vi "App - analyze RUS V6.vi"() -> ()   [LabVIEW 2021] (continued)
"lorentzian"={"A (VHz)"=0.0, "ω (Hz)"=0.0, "Γ (Hz)"=0.0, "φ (rad)"=0.0, "Q"=0.0, "Norm  Ampl"=0.0, "z∞ (V)"=0.0+0.0i, "4corners"={"z (-pi/2)"=0.0+0.0i, "z(inf)"=0.0+0.0i, "z (pi/2)"=0.0+0.0i, "z center"=0.0+0.0i, "z(0)"=0.0+0.0i, "radius"=0.0}}, "timestamp(min)"=1735.7333333343267, "timestamp"=timestamp(3493831965 s since 1904-01-01), "Magn Field(T)"=0.0}, {"temperature"=32.55, "lorentzian"={"A (VHz)"=0.0, "ω (Hz)"=0.0, "Γ (Hz)"=0.0, "φ (rad)"=0.0, "Q"=0.0, "Norm  Ampl"=0.0, "z∞ (V)"=0.0+0.0i, "4corners"={"z (-pi/2)"=0.0+0.0i, "z(inf)"=0.0+0.0i, "z (pi/2)"=0.0+0.0i, "z center"=0.0+0.0i, "z(0)"=0.0+0.0i, "radius"=0.0}}, "timestamp(min)"=1737.0500000044703, "timestamp"=timestamp(3493832044 s since 1904-01-01), "Magn Field(T)"=0.0}, {"temperature"=32.462, "lorentzian"={"A (VHz)"=0.0, "ω (Hz)"=0.0, "Γ (Hz)"=0.0, "φ (rad)"=0.0, "Q"=0.0, "Norm  Ampl"=0.0, "z∞ (V)"=0.0+0.0i, "4corners"={"z (-pi/2)"=0.0+0.0i, "z(inf)"=0.0+0.0i, "z (pi/2)"=0.0+0.0i, "z center"=0.0+0.0i, "z(0)"=0.0+0.0i, "radius"=0.0}}, "timestamp(min)"=1738.3666666671634, "timestamp"=timestamp(3493832123 s since 1904-01-01), "Magn Field(T)"=0.0}, {"temperature"=32.371, "lorentzian"={"A (VHz)"=0.0, "ω (Hz)"=0.0, "Γ (Hz)"=0.0, "φ (rad)"=0.0, "Q"=0.0, "Norm  Ampl"=0.0, "z∞ (V)"=0.0+0.0i, "4corners"={"z (-pi/2)"=0.0+0.0i, "z(inf)"=0.0+0.0i, "z (pi/2)"=0.0+0.0i, "z center"=0.0+0.0i, "z(0)"=0.0+0.0i, "radius"=0.0}}, "timestamp(min)"=1739.7000000029802, "timestamp"=timestamp(3493832203 s since 1904-01-01), "Magn Field(T)"=0.0}, {"temperature"=32.282, "lorentzian"={"A (VHz)"=0.0, "ω (Hz)"=0.0, "Γ (Hz)"=0.0, "φ (rad)"=0.0, "Q"=0.0, "Norm  Ampl"=0.0, "z∞ (V)"=0.0+0.0i, "4corners"={"z (-pi/2)"=0.0+0.0i, "z(inf)"=0.0+0.0i, "z (pi/2)"=0.0+0.0i, "z center"=0.0+0.0i, "z(0)"=0.0+0.0i, "radius"=0.0}}, "timestamp(min)"=1741.0166666656733, "timestamp"=timestamp(3493832282 s since 1904-01-01), "Magn Field(T)"=0.0}, {"temperature"=32.189, "lorentzian"={"A (VHz)"=0.0, "ω (Hz)"=0.0, "Γ (Hz)"=0.0, "φ (rad)"=0.0, "Q"=0.0, "Norm  Ampl"=0.0, "z∞ (V)"=0.0+0.0i, "4corners"={"z (-pi/2)"=0.0+0.0i, "z(inf)"=0.0+0.0i, "z (pi/2)"=0.0+0.0i, "z center"=0.0+0.0i, "z(0)"=0.0+0.0i, "radius"=0.0}}, "timestamp(min)"=1742.3500000014901, "timestamp"=timestamp(3493832362 s since 1904-01-01), "Magn Field(T)"=0.0}, {"temperature"=32.102, "lorentzian"={"A (VHz)"=0.0, "ω (Hz)"=0.0, "Γ (Hz)"=0.0, "φ (rad)"=0.0, "Q"=0.0, "Norm  Ampl"=0.0, "z∞ (V)"=0.0+0.0i, "4corners"={"z (-pi/2)"=0.0+0.0i, "z(inf)"=0.0+0.0i, "z (pi/2)"=0.0+0.0i, "z center"=0.0+0.0i, "z(0)"=0.0+0.0i, "radius"=0.0}}, "timestamp(min)"=1743.6666666641831, "timestamp"=timestamp(3493832441 s since 1904-01-01), "Magn Field(T)"=0.0}, {"temperature"=32.008, "lorentzian"={"A (VHz)"=0.0, "ω (Hz)"=0.0, "Γ (Hz)"=0.0, "φ (rad)"=0.0, "Q"=0.0, "Norm  Ampl"=0.0, "z∞ (V)"=0.0+0.0i, "4corners"={"z (-pi/2)"=0.0+0.0i, "z(inf)"=0.0+0.0i, "z (pi/2)"=0.0+0.0i, "z center"=0.0+0.0i, "z(0)"=0.0+0.0i, "radius"=0.0}}, "timestamp(min)"=1744.9833333343267, "timestamp"=timestamp(3493832520 s since 1904-01-01), "Magn Field(T)"=0.0}, {"temperature"=31.925, "lorentzian"={"A (VHz)"=0.0, "ω (Hz)"=0.0, "Γ (Hz)"=0.0, "φ (rad)"=0.0, "Q"=0.0, "Norm  Ampl"=0.0, "z∞ (V)"=0.0+0.0i, "4corners"={"z (-pi/2)"=0.0+0.0i, "z(inf)"=0.0+0.0i, "z (pi/2)"=0.0+0.0i, "z center"=0.0+0.0i, "z(0)"=0.0+0.0i, "radius"=0.0}}, "timestamp(min)"=1746.3166666701436, "timestamp"=timestamp(3493832600 s since 1904-01-01), "Magn Field(T)"=0.0}, {"temperature"=31.83, "lorentzian"={"A (VHz)"=0.0, "ω (Hz)"=0.0, "Γ (Hz)"=0.0, "φ (rad)"=0.0, "Q"=0.0, "Norm  Ampl"=0.0, "z∞ (V)"=0.0+0.0i, "4corners"={"z (-pi/2)"=0.0+0.0i, "z(inf)"=0.0+0.0i, "z (pi/2)"=0.0+0.0i, "z center"=0.0+0.0i, "z(0)"=0.0+0.0i, "radius"=0.0}}, "timestamp(min)"=1747.6333333328366, "timestamp"=timestamp(3493832679 s since 1904-01-01), "Magn Field(T)"=0.0}, {"temperature"=31.738, "lorentzian"={"A (VHz)"=0.0, "ω (Hz)"=0.0, "Γ (Hz)"=0.0, "φ (rad)"=0.0, "Q"=0.0, "Norm  Ampl"=0.0, "z∞ (V)"=0.0+0.0i, "4corners"={"z (-pi/2)"=0.0+0.0i, "z(inf)"=0.0+0.0i, "z (pi/2)"=0.0+0.0i, "z center"=0.0+0.0i, "z(0)"=0.0+0.0i, "radius"=0.0}}, "timestamp(min)"=1748.9500000029802, "timestamp"=timestamp(3493832758 s since 1904-01-01), "Magn Field(T)"=0.0}, {"temperature"=31.653, "lorentzian"={"A (VHz)"=0.0, "ω (Hz)"=0.0, "Γ (Hz)"=0.0, "φ (rad)"=0.0, "Q"=0.0, "Norm  Ampl"=0.0, "z∞ (V)"=0.0+0.0i, "4corners"={"z (-pi/2)"=0.0+0.0i, "z(inf)"=0.0+0.0i, "z (pi/2)"=0.0+0.0i, "z center"=0.0+0.0i, "z(0)"=0.0+0.0i, "radius"=0.0}}, "timestamp(min)"=1750.2833333313465, "timestamp"=timestamp(3493832838 s since 1904-01-01), "Magn Field(T)"=0.0}, {"temperature"=31.556, "lorentzian"={"A (VHz)"=0.0, "ω (Hz)"=0.0, "Γ (Hz)"=0.0, "φ (rad)"=0.0, "Q"=0.0, "Norm  Ampl"=0.0, "z∞ (V)"=0.0+0.0i, "4corners"={"z (-pi/2)"=0.0+0.0i, "z(inf)"=0.0+0.0i, "z (pi/2)"=0.0+0.0i, "z center"=0.0+0.0i, "z(0)"=0.0+0.0i, "radius"=0.0}}, "timestamp(min)"=1751.6000000014901, "timestamp"=timestamp(3493832917 s since 1904-01-01), "Magn Field(T)"=0.0}, {"temperature"=31.463, "lorentzian"={"A (VHz)"=0.0, "ω (Hz)"=0.0, "Γ (Hz)"=0.0, "φ (rad)"=0.0, "Q"=0.0, "Norm  Ampl"=0.0, "z∞ (V)"=0.0+0.0i, "4corners"={"z (-pi/2)"=0.0+0.0i, "z(inf)"=0.0+0.0i, "z (pi/2)"=0.0+0.0i, "z center"=0.0+0.0i, "z(0)"=0.0+0.0i, "radius"=0.0}}, "timestamp(min)"=1752.933333337307, "timestamp"=timestamp(3493832997 s since 1904-01-01), "Magn Field(T)"=0.0}, {"temperature"=31.383, "lorentzian"={"A (VHz)"=0.0, "ω (Hz)"=0.0, "Γ (Hz)"=0.0, "φ (rad)"=0.0, "Q"=0.0, "Norm  Ampl"=0.0, "z∞ (V)"=0.0+0.0i, "4corners"={"z (-pi/2)"=0.0+0.0i, "z(inf)"=0.0+0.0i, "z (pi/2)"=0.0+0.0i, "z center"=0.0+0.0i, "z(0)"=0.0+0.0i, "radius"=0.0}}, "timestamp(min)"=1754.25, "timestamp"=timestamp(3493833076 s since 1904-01-01), "Magn Field(T)"=0.0}, {"temperature"=31.282, "lorentzian"={"A (VHz)"=0.0, "ω (Hz)"=0.0, "Γ (Hz)"=0.0, "φ (rad)"=0.0, "Q"=0.0, "Norm  Ampl"=0.0, "z∞ (V)"=0.0+0.0i, "4corners"={"z (-pi/2)"=0.0+0.0i, "z(inf)"=0.0+0.0i, "z (pi/2)"=0.0+0.0i, "z center"=0.0+0.0i, "z(0)"=0.0+0.0i, "radius"=0.0}}, "timestamp(min)"=1755.5666666701436, "timestamp"=timestamp(3493833155 s since 1904-01-01), "Magn Field(T)"=0.0}, {"temperature"=31.196, "lorentzian"={"A (VHz)"=0.0, "ω (Hz)"=0.0, "Γ (Hz)"=0.0, "φ (rad)"=0.0, "Q"=0.0, "Norm  Ampl"=0.0, "z∞ (V)"=0.0+0.0i, "4corners"={"z (-pi/2)"=0.0+0.0i, "z(inf)"=0.0+0.0i, "z (pi/2)"=0.0+0.0i, "z center"=0.0+0.0i, "z(0)"=0.0+0.0i, "radius"=0.0}}, "timestamp(min)"=1756.8999999985099, "timestamp"=timestamp(3493833235 s since 1904-01-01), "Magn Field(T)"=0.0}, {"temperature"=31.111, "lorentzian"={"A (VHz)"=0.0, "ω (Hz)"=0.0, "Γ (Hz)"=0.0, "φ (rad)"=0.0, "Q"=0.0, "Norm  Ampl"=0.0, "z∞ (V)"=0.0+0.0i, "4corners"={"z (-pi/2)"=0.0+0.0i, "z(inf)"=0.0+0.0i, "z (pi/2)"=0.0+0.0i, "z center"=0.0+0.0i, "z(0)"=0.0+0.0i, "radius"=0.0}}, "timestamp(min)"=1758.2166666686535, "timestamp"=timestamp(3493833314 s since 1904-01-01), "Magn Field(T)"=0.0}, {"temperature"=31.006, "lorentzian"={"A (VHz)"=0.0, "ω (Hz)"=0.0, "Γ (Hz)"=0.0, "φ (rad)"=0.0, "Q"=0.0, "Norm  Ampl"=0.0, "z∞ (V)"=0.0+0.0i, "4corners"={"z (-pi/2)"=0.0+0.0i, "z(inf)"=0.0+0.0i, "z (pi/2)"=0.0+0.0i, "z center"=0.0+0.0i, "z(0)"=0.0+0.0i, "radius"=0.0}}, "timestamp(min)"=1759.5333333313465, "timestamp"=timestamp(3493833393 s since 1904-01-01), "Magn Field(T)"=0.0}, {"temperature"=30.926, "lorentzian"={"A (VHz)"=0.0, "ω (Hz)"=0.0, "Γ (Hz)"=0.0, "φ (rad)"=0.0, "Q"=0.0, "Norm  Ampl"=0.0, "z∞ (V)"=0.0+0.0i, "4corners"={"z (-pi/2)"=0.0+0.0i, "z(inf)"=0.0+0.0i, "z (pi/2)"=0.0+0.0i, "z center"=0.0+0.0i, "z(0)"=0.0+0.0i, "radius"=0.0}}, "timestamp(min)"=1760.8666666671634, "timestamp"=timestamp(3493833473 s since 1904-01-01), "Magn Field(T)"=0.0}, {"temperature"=30.834, "lorentzian"={"A (VHz)"=0.0, "ω (Hz)"=0.0, "Γ (Hz)"=0.0, "φ (rad)"=0.0, "Q"=0.0, "Norm  Ampl"=0.0, "z∞ (V)"=0.0+0.0i, "4corners"={"z (-pi/2)"=0.0+0.0i, "z(inf)"=0.0+0.0i, "z (pi/2)"=0.0+0.0i, "z center"=0.0+0.0i, "z(0)"=0.0+0.0i, "radius"=0.0}}, "timestamp(min)"=1762.183333337307, "timestamp"=timestamp(3493833552 s since 1904-01-01), "Magn Field(T)"=0.0}, {"temperature"=30.738, "lorentzian"={"A (VHz)"=0.0, "ω (Hz)"=0.0, "Γ (Hz)"=0.0, "φ (rad)"=0.0, "Q"=0.0, "Norm  Ampl"=0.0, "z∞ (V)"=0.0+0.0i, "4corners"={"z (-pi/2)"=0.0+0.0i, "z(inf)"=0.0+0.0i, "z (pi/2)"=0.0+0.0i, "z center"=0.0+0.0i, "z(0)"=0.0+0.0i, "radius"=0.0}}, "timestamp(min)"=1763.5166666656733, "timestamp"=timestamp(3493833632 s since 1904-01-01), "Magn Field(T)"=0.0}, {"temperature"=30.648, "lorentzian"={"A (VHz)"=0.0, "ω (Hz)"=0.0, "Γ (Hz)"=0.0, "φ (rad)"=0.0, "Q"=0.0, "Norm  Ampl"=0.0, "z∞ (V)"=0.0+0.0i, "4corners"={"z (-pi/2)"=0.0+0.0i, "z(inf)"=0.0+0.0i, "z (pi/2)"=0.0+0.0i, "z center"=0.0+0.0i, "z(0)"=0.0+0.0i, "radius"=0.0}}, "timestamp(min)"=1764.8333333358169, "timestamp"=timestamp(3493833711 s since 1904-01-01), "Magn Field(T)"=0.0}, {"temperature"=30.563, "lorentzian"={"A (VHz)"=0.0, "ω (Hz)"=0.0, "Γ (Hz)"=0.0, "φ (rad)"=0.0, "Q"=0.0, "Norm  Ampl"=0.0, "z∞ (V)"=0.0+0.0i, "4corners"={"z (-pi/2)"=0.0+0.0i, "z(inf)"=0.0+0.0i, "z (pi/2)"=0.0+0.0i, "z center"=0.0+0.0i, "z(0)"=0.0+0.0i, "radius"=0.0}}, "timestamp(min)"=1766.1499999985099, "timestamp"=timestamp(3493833790 s since 1904-01-01), "Magn Field(T)"=0.0}, {"temperature"=30.467, "lorentzian"={"A (VHz)"=0.0, "ω (Hz)"=0.0, "Γ (Hz)"=0.0, "φ (rad)"=0.0, "Q"=0.0, "Norm  Ampl"=0.0, "z∞ (V)"=0.0+0.0i, "4corners"={"z (-pi/2)"=0.0+0.0i, "z(inf)"=0.0+0.0i, "z (pi/2)"=0.0+0.0i, "z center"=0.0+0.0i, "z(0)"=0.0+0.0i, "radius"=0.0}}, "timestamp(min)"=1767.4833333343267, "timestamp"=timestamp(3493833870 s since 1904-01-01), "Magn Field(T)"=0.0}, {"temperature"=30.376, "lorentzian"={"A (VHz)"=0.0, "ω (Hz)"=0.0, "Γ (Hz)"=0.0, "φ (rad)"=0.0, "Q"=0.0, "Norm  Ampl"=0.0, "z∞ (V)"=0.0+0.0i, "4corners"={"z (-pi/2)"=0.0+0.0i, "z(inf)"=0.0+0.0i, "z (pi/2)"=0.0+0.0i, "z center"=0.0+0.0i, "z(0)"=0.0+0.0i, "radius"=0.0}}, "timestamp(min)"=1768.8000000044703, "timestamp"=timestamp(3493833949 s since 1904-01-01), "Magn Field(T)"=0.0}, {"temperature"=30.285, "lorentzian"={"A (VHz)"=0.0, "ω (Hz)"=0.0, "Γ (Hz)"=0.0, "φ (rad)"=0.0, "Q"=0.0, "Norm  Ampl"=0.0, "z∞ (V)"=0.0+0.0i, "4corners"={"z (-pi/2)"=0.0+0.0i, "z(inf)"=0.0+0.0i, "z (pi/2)"=0.0+0.0i, "z center"=0.0+0.0i, "z(0)"=0.0+0.0i, "radius"=0.0}}, "timestamp(min)"=1770.1333333328366, "timestamp"=timestamp(3493834029 s since 1904-01-01), "Magn Field(T)"=0.0}, {"temperature"=30.196, "lorentzian"={"A (VHz)"=0.0, "ω (Hz)"=0.0, "Γ (Hz)"=0.0, "φ (rad)"=0.0, "Q"=0.0, "Norm  Ampl"=0.0, "z∞ (V)"=0.0+0.0i, "4corners"={"z (-pi/2)"=0.0+0.0i, "z(inf)"=0.0+0.0i, "z (pi/2)"=0.0+0.0i, "z center"=0.0+0.0i, "z(0)"=0.0+0.0i, "radius"=0.0}}, "timestamp(min)"=1771.4500000029802, "timestamp"=timestamp(3493834108 s since 1904-01-01), "Magn Field(T)"=0.0}, {"temperature"=30.104, "lorentzian"={"A (VHz)"=0.0, "ω (Hz)"=0.0, "Γ (Hz)"=0.0, "φ (rad)"=0.0, "Q"=0.0, "Norm  Ampl"=0.0, "z∞ (V)"=0.0+0.0i, "4corners"={"z (-pi/2)"=0.0+0.0i, "z(inf)"=0.0+0.0i, "z (pi/2)"=0.0+0.0i, "z center"=0.0+0.0i, "z(0)"=0.0+0.0i, "radius"=0.0}}, "timestamp(min)"=1772.7666666656733, "timestamp"=timestamp(3493834187 s since 1904-01-01), "Magn Field(T)"=0.0}, {"temperature"=30.009, "lorentzian"={"A (VHz)"=0.0, "ω (Hz)"=0.0, "Γ (Hz)"=0.0, "φ (rad)"=0.0, "Q"=0.0, "Norm  Ampl"=0.0, "z∞ (V)"=0.0+0.0i, "4corners"={"z (-pi/2)"=0.0+0.0i, "z(inf)"=0.0+0.0i, "z (pi/2)"=0.0+0.0i, "z center"=0.0+0.0i, "z(0)"=0.0+0.0i, "radius"=0.0}}, "timestamp(min)"=1774.1000000014901, "timestamp"=timestamp(3493834267 s since 1904-01-01), "Magn Field(T)"=0.0}, {"temperature"=29.914, "lorentzian"={"A (VHz)"=0.0, "ω (Hz)"=0.0, "Γ (Hz)"=0.0, "φ (rad)"=0.0, "Q"=0.0, "Norm  Ampl"=0.0, "z∞ (V)"=0.0+0.0i, "4corners"={"z (-pi/2)"=0.0+0.0i, "z(inf)"=0.0+0.0i, "z (pi/2)"=0.0+0.0i, "z center"=0.0+0.0i, "z(0)"=0.0+0.0i, "radius"=0.0}}, "timestamp(min)"=1775.4166666641831, "timestamp"=timestamp(3493834346 s since 1904-01-01), "Magn Field(T)"=0.0}, {"temperature"=29.832, "lorentzian"={"A (VHz)"=0.0, "ω (Hz)"=0.0, "Γ (Hz)"=0.0, "φ (rad)"=0.0, "Q"=0.0, "Norm  Ampl"=0.0, "z∞ (V)"=0.0+0.0i, "4corners"={"z (-pi/2)"=0.0+0.0i, "z(inf)"=0.0+0.0i, "z (pi/2)"=0.0+0.0i, "z center"=0.0+0.0i, "z(0)"=0.0+0.0i, "radius"=0.0}}, "timestamp(min)"=1776.7333333343267, "timestamp"=timestamp(3493834425 s since 1904-01-01), "Magn Field(T)"=0.0}, {"temperature"=29.737, "lorentzian"={"A (VHz)"=0.0, "ω (Hz)"=0.0, "Γ (Hz)"=0.0, "φ (rad)"=0.0, "Q"=0.0, "Norm  Ampl"=0.0, "z∞ (V)"=0.0+0.0i, "4corners"={"z (-pi/2)"=0.0+0.0i, "z(inf)"=0.0+0.0i, "z (pi/2)"=0.0+0.0i, "z center"=0.0+0.0i, "z(0)"=0.0+0.0i, "radius"=0.0}}, "timestamp(min)"=1778.0666666701436, "timestamp"=timestamp(3493834505 s since 1904-01-01), "Magn Field(T)"=0.0}, {"temperature"=29.637, "lorentzian"={"A (VHz)"=0.0, "ω (Hz)"=0.0, "Γ (Hz)"=0.0, "φ (rad)"=0.0, "Q"=0.0, "Norm  Ampl"=0.0, "z∞ (V)"=0.0+0.0i, "4corners"={"z (-pi/2)"=0.0+0.0i, "z(inf)"=0.0+0.0i, "z (pi/2)"=0.0+0.0i, "z center"=0.0+0.0i, "z(0)"=0.0+0.0i, "radius"=0.0}}, "timestamp(min)"=1779.3833333328366, "timestamp"=timestamp(3493834584 s since 1904-01-01), "Magn Field(T)"=0.0}, {"temperature"=29.553, "lorentzian"={"A (VHz)"=0.0, "ω (Hz)"=0.0, "Γ (Hz)"=0.0, "φ (rad)"=0.0, "Q"=0.0, "Norm  Ampl"=0.0, "z∞ (V)"=0.0+0.0i, "4corners"={"z (-pi/2)"=0.0+0.0i, "z(inf)"=0.0+0.0i, "z (pi/2)"=0.0+0.0i, "z center"=0.0+0.0i, "z(0)"=0.0+0.0i, "radius"=0.0}}, "timestamp(min)"=1780.7166666686535, "timestamp"=timestamp(3493834664 s since 1904-01-01), "Magn Field(T)"=0.0}, {"temperature"=29.453, "lorentzian"={"A (VHz)"=0.0, "ω (Hz)"=0.0, "Γ (Hz)"=0.0, "φ (rad)"=0.0, "Q"=0.0, "Norm  Ampl"=0.0, "z∞ (V)"=0.0+0.0i, "4corners"={"z (-pi/2)"=0.0+0.0i, "z(inf)"=0.0+0.0i, "z (pi/2)"=0.0+0.0i, "z center"=0.0+0.0i, "z(0)"=0.0+0.0i, "radius"=0.0}}, "timestamp(min)"=1782.0333333313465, "timestamp"=timestamp(3493834743 s since 1904-01-01), "Magn Field(T)"=0.0}, {"temperature"=29.362, "lorentzian"={"A (VHz)"=0.0, "ω (Hz)"=0.0, "Γ (Hz)"=0.0, "φ (rad)"=0.0, "Q"=0.0, "Norm  Ampl"=0.0, "z∞ (V)"=0.0+0.0i, "4corners"={"z (-pi/2)"=0.0+0.0i, "z(inf)"=0.0+0.0i, "z (pi/2)"=0.0+0.0i, "z center"=0.0+0.0i, "z(0)"=0.0+0.0i, "radius"=0.0}}, "timestamp(min)"=1783.3500000014901, "timestamp"=timestamp(3493834822 s since 1904-01-01), "Magn Field(T)"=0.0}, {"temperature"=29.272, "lorentzian"={"A (VHz)"=0.0, "ω (Hz)"=0.0, "Γ (Hz)"=0.0, "φ (rad)"=0.0, "Q"=0.0, "Norm  Ampl"=0.0, "z∞ (V)"=0.0+0.0i, "4corners"={"z (-pi/2)"=0.0+0.0i, "z(inf)"=0.0+0.0i, "z (pi/2)"=0.0+0.0i, "z center"=0.0+0.0i, "z(0)"=0.0+0.0i, "radius"=0.0}}, "timestamp(min)"=1784.683333337307, "timestamp"=timestamp(3493834902 s since 1904-01-01), "Magn Field(T)"=0.0}, {"temperature"=29.18, "lorentzian"={"A (VHz)"=0.0, "ω (Hz)"=0.0, "Γ (Hz)"=0.0, "φ (rad)"=0.0, "Q"=0.0, "Norm  Ampl"=0.0, "z∞ (V)"=0.0+0.0i, "4corners"={"z (-pi/2)"=0.0+0.0i, "z(inf)"=0.0+0.0i, "z (pi/2)"=0.0+0.0i, "z center"=0.0+0.0i, "z(0)"=0.0+0.0i, "radius"=0.0}}, "timestamp(min)"=1786.0, "timestamp"=timestamp(3493834981 s since 1904-01-01), "Magn Field(T)"=0.0}, {"temperature"=29.085, "lorentzian"={"A (VHz)"=0.0, "ω (Hz)"=0.0, "Γ (Hz)"=0.0, "φ (rad)"=0.0, "Q"=0.0, "Norm  Ampl"=0.0, "z∞ (V)"=0.0+0.0i, "4corners"={"z (-pi/2)"=0.0+0.0i, "z(inf)"=0.0+0.0i, "z (pi/2)"=0.0+0.0i, "z center"=0.0+0.0i, "z(0)"=0.0+0.0i, "radius"=0.0}}, "timestamp(min)"=1787.3333333358169, "timestamp"=timestamp(3493835061 s since 1904-01-01), "Magn Field(T)"=0.0}, {"temperature"=28.992, "lorentzian"={"A (VHz)"=0.0, "ω (Hz)"=0.0, "Γ (Hz)"=0.0, "φ (rad)"=0.0, "Q"=0.0, "Norm  Ampl"=0.0, "z∞ (V)"=0.0+0.0i, "4corners"={"z (-pi/2)"=0.0+0.0i, "z(inf)"=0.0+0.0i, "z (pi/2)"=0.0+0.0i, "z center"=0.0+0.0i, "z(0)"=0.0+0.0i, "radius"=0.0}}, "timestamp(min)"=1788.6499999985099, "timestamp"=timestamp(3493835140 s since 1904-01-01), "Magn Field(T)"=0.0}, {"temperature"=28.892, "lorentzian"={"A (VHz)"=0.0, "ω (Hz)"=0.0, "Γ (Hz)"=0.0, "φ (rad)"=0.0, "Q"=0.0, "Norm  Ampl"=0.0, "z∞ (V)"=0.0+0.0i, "4corners"={"z (-pi/2)"=0.0+0.0i, "z(inf)"=0.0+0.0i, "z (pi/2)"=0.0+0.0i, "z center"=0.0+0.0i, "z(0)"=0.0+0.0i, "radius"=0.0}}, "timestamp(min)"=1789.9666666686535, "timestamp"=timestamp(3493835219 s since 1904-01-01), "Magn Field(T)"=0.0}, {"temperature"=28.803, "lorentzian"={"A (VHz)"=0.0, "ω (Hz)"=0.0, "Γ (Hz)"=0.0, "φ (rad)"=0.0, "Q"=0.0, "Norm  Ampl"=0.0, "z∞ (V)"=0.0+0.0i, "4corners"={"z (-pi/2)"=0.0+0.0i, "z(inf)"=0.0+0.0i, "z (pi/2)"=0.0+0.0i, "z center"=0.0+0.0i, "z(0)"=0.0+0.0i, "radius"=0.0}}, "timestamp(min)"=1791.3000000044703, "timestamp"=timestamp(3493835299 s since 1904-01-01), "Magn Field(T)"=0.0}, {"temperature"=28.71, "lorentzian"={"A (VHz)"=0.0, "ω (Hz)"=0.0, "Γ (Hz)"=0.0, "φ (rad)"=0.0, "Q"=0.0, "Norm  Ampl"=0.0, "z∞ (V)"=0.0+0.0i, "4corners"={"z (-pi/2)"=0.0+0.0i, "z(inf)"=0.0+0.0i, "z (pi/2)"=0.0+0.0i, "z center"=0.0+0.0i, "z(0)"=0.0+0.0i, "radius"=0.0}}, "timestamp(min)"=1792.6166666671634, "timestamp"=timestamp(3493835378 s since 1904-01-01), "Magn Field(T)"=0.0}, {"temperature"=28.614, "lorentzian"={"A (VHz)"=0.0, "ω (Hz)"=0.0, "Γ (Hz)"=0.0, "φ (rad)"=0.0, "Q"=0.0, "Norm  Ampl"=0.0, "z∞ (V)"=0.0+0.0i, "4corners"={"z (-pi/2)"=0.0+0.0i, "z(inf)"=0.0+0.0i, "z (pi/2)"=0.0+0.0i, "z center"=0.0+0.0i, "z(0)"=0.0+0.0i, "radius"=0.0}}, "timestamp(min)"=1793.933333337307, "timestamp"=timestamp(3493835457 s since 1904-01-01), "Magn Field(T)"=0.0}, {"temperature"=28.52, "lorentzian"={"A (VHz)"=0.0, "ω (Hz)"=0.0, "Γ (Hz)"=0.0, "φ (rad)"=0.0, "Q"=0.0, "Norm  Ampl"=0.0, "z∞ (V)"=0.0+0.0i, "4corners"={"z (-pi/2)"=0.0+0.0i, "z(inf)"=0.0+0.0i, "z (pi/2)"=0.0+0.0i, "z center"=0.0+0.0i, "z(0)"=0.0+0.0i, "radius"=0.0}}, "timestamp(min)"=1795.2666666656733, "timestamp"=timestamp(3493835537 s since 1904-01-01), "Magn Field(T)"=0.0}, {"temperature"=28.426, "lorentzian"={"A (VHz)"=0.0, "ω (Hz)"=0.0, "Γ (Hz)"=0.0, "φ (rad)"=0.0, "Q"=0.0, "Norm  Ampl"=0.0, "z∞ (V)"=0.0+0.0i, "4corners"={"z (-pi/2)"=0.0+0.0i, "z(inf)"=0.0+0.0i, "z (pi/2)"=0.0+0.0i, "z center"=0.0+0.0i, "z(0)"=0.0+0.0i, "radius"=0.0}}, "timestamp(min)"=1796.5833333358169, "timestamp"=timestamp(3493835616 s since 1904-01-01), "Magn Field(T)"=0.0}, {"temperature"=28.336, "lorentzian"={"A (VHz)"=0.0, "ω (Hz)"=0.0, "Γ (Hz)"=0.0, "φ (rad)"=0.0, "Q"=0.0, "Norm  Ampl"=0.0, "z∞ (V)"=0.0+0.0i, "4corners"={"z (-pi/2)"=0.0+0.0i, "z(inf)"=0.0+0.0i, "z (pi/2)"=0.0+0.0i, "z center"=0.0+0.0i, "z(0)"=0.0+0.0i, "radius"=0.0}}, "timestamp(min)"=1797.9166666641831, "timestamp"=timestamp(3493835696 s since 1904-01-01), "Magn Field(T)"=0.0}, {"temperature"=28.239, "lorentzian"={"A (VHz)"=0.0, "ω (Hz)"=0.0, "Γ (Hz)"=0.0, "φ (rad)"=0.0, "Q"=0.0, "Norm  Ampl"=0.0, "z∞ (V)"=0.0+0.0i, "4corners"={"z (-pi/2)"=0.0+0.0i, "z(inf)"=0.0+0.0i, "z (pi/2)"=0.0+0.0i, "z center"=0.0+0.0i, "z(0)"=0.0+0.0i, "radius"=0.0}}, "timestamp(min)"=1799.2333333343267, "timestamp"=timestamp(3493835775 s since 1904-01-01), "Magn Field(T)"=0.0}, {"temperature"=28.151, "lorentzian"={"A (VHz)"=0.0, "ω (Hz)"=0.0, "Γ (Hz)"=0.0, "φ (rad)"=0.0, "Q"=0.0, "Norm  Ampl"=0.0, "z∞ (V)"=0.0+0.0i, "4corners"={"z (-pi/2)"=0.0+0.0i, "z(inf)"=0.0+0.0i, "z (pi/2)"=0.0+0.0i, "z center"=0.0+0.0i, "z(0)"=0.0+0.0i, "radius"=0.0}}, "timestamp(min)"=1800.5500000044703, "timestamp"=timestamp(3493835854 s since 1904-01-01), "Magn Field(T)"=0.0}, {"temperature"=28.051, "lorentzian"={"A (VHz)"=0.0, "ω (Hz)"=0.0, "Γ (Hz)"=0.0, "φ (rad)"=0.0, "Q"=0.0, "Norm  Ampl"=0.0, "z∞ (V)"=0.0+0.0i, "4corners"={"z (-pi/2)"=0.0+0.0i, "z(inf)"=0.0+0.0i, "z (pi/2)"=0.0+0.0i, "z center"=0.0+0.0i, "z(0)"=0.0+0.0i, "radius"=0.0}}, "timestamp(min)"=1801.8833333328366, "timestamp"=timestamp(3493835934 s since 1904-01-01), "Magn Field(T)"=0.0}, {"temperature"=27.959, "lorentzian"={"A (VHz)"=0.0, "ω (Hz)"=0.0, "Γ (Hz)"=0.0, "φ (rad)"=0.0, "Q"=0.0, "Norm  Ampl"=0.0, "z∞ (V)"=0.0+0.0i, "4corners"={"z (-pi/2)"=0.0+0.0i, "z(inf)"=0.0+0.0i, "z (pi/2)"=0.0+0.0i, "z center"=0.0+0.0i, "z(0)"=0.0+0.0i, "radius"=0.0}}, "timestamp(min)"=1803.2000000029802, "timestamp"=timestamp(3493836013 s since 1904-01-01), "Magn Field(T)"=0.0}, {"temperature"=27.87, "lorentzian"={"A (VHz)"=0.0, "ω (Hz)"=0.0, "Γ (Hz)"=0.0, "φ (rad)"=0.0, "Q"=0.0, "Norm  Ampl"=0.0, "z∞ (V)"=0.0+0.0i, "4corners"={"z (-pi/2)"=0.0+0.0i, "z(inf)"=0.0+0.0i, "z (pi/2)"=0.0+0.0i, "z center"=0.0+0.0i, "z(0)"=0.0+0.0i, "radius"=0.0}}, "timestamp(min)"=1804.5166666656733, "timestamp"=timestamp(3493836092 s since 1904-01-01), "Magn Field(T)"=0.0}, {"temperature"=27.768, "lorentzian"={"A (VHz)"=0.0, "ω (Hz)"=0.0, "Γ (Hz)"=0.0, "φ (rad)"=0.0, "Q"=0.0, "Norm  Ampl"=0.0, "z∞ (V)"=0.0+0.0i, "4corners"={"z (-pi/2)"=0.0+0.0i, "z(inf)"=0.0+0.0i, "z (pi/2)"=0.0+0.0i, "z center"=0.0+0.0i, "z(0)"=0.0+0.0i, "radius"=0.0}}, "timestamp(min)"=1805.8500000014901, "timestamp"=timestamp(3493836172 s since 1904-01-01), "Magn Field(T)"=0.0}, {"temperature"=27.675, "lorentzian"={"A (VHz)"=0.0, "ω (Hz)"=0.0, "Γ (Hz)"=0.0, "φ (rad)"=0.0, "Q"=0.0, "Norm  Ampl"=0.0, "z∞ (V)"=0.0+0.0i, "4corners"={"z (-pi/2)"=0.0+0.0i, "z(inf)"=0.0+0.0i, "z (pi/2)"=0.0+0.0i, "z center"=0.0+0.0i, "z(0)"=0.0+0.0i, "radius"=0.0}}, "timestamp(min)"=1807.1666666641831, "timestamp"=timestamp(3493836251 s since 1904-01-01), "Magn Field(T)"=0.0}, {"temperature"=27.583, "lorentzian"={"A (VHz)"=0.0, "ω (Hz)"=0.0, "Γ (Hz)"=0.0, "φ (rad)"=0.0, "Q"=0.0, "Norm  Ampl"=0.0, "z∞ (V)"=0.0+0.0i, "4corners"={"z (-pi/2)"=0.0+0.0i, "z(inf)"=0.0+0.0i, "z (pi/2)"=0.0+0.0i, "z center"=0.0+0.0i, "z(0)"=0.0+0.0i, "radius"=0.0}}, "timestamp(min)"=1808.5, "timestamp"=timestamp(3493836331 s since 1904-01-01), "Magn Field(T)"=0.0}, {"temperature"=27.483, "lorentzian"={"A (VHz)"=0.0, "ω (Hz)"=0.0, "Γ (Hz)"=0.0, "φ (rad)"=0.0, "Q"=0.0, "Norm  Ampl"=0.0, "z∞ (V)"=0.0+0.0i, "4corners"={"z (-pi/2)"=0.0+0.0i, "z(inf)"=0.0+0.0i, "z (pi/2)"=0.0+0.0i, "z center"=0.0+0.0i, "z(0)"=0.0+0.0i, "radius"=0.0}}, "timestamp(min)"=1809.8166666701436, "timestamp"=timestamp(3493836410 s since 1904-01-01), "Magn Field(T)"=0.0}, {"temperature"=27.396, "lorentzian"={"A (VHz)"=0.0, "ω (Hz)"=0.0, "Γ (Hz)"=0.0, "φ (rad)"=0.0, "Q"=0.0, "Norm  Ampl"=0.0, "z∞ (V)"=0.0+0.0i, "4corners"={"z (-pi/2)"=0.0+0.0i, "z(inf)"=0.0+0.0i, "z (pi/2)"=0.0+0.0i, "z center"=0.0+0.0i, "z(0)"=0.0+0.0i, "radius"=0.0}}, "timestamp(min)"=1811.1333333328366, "timestamp"=timestamp(3493836489 s since 1904-01-01), "Magn Field(T)"=0.0}, {"temperature"=27.297, "lorentzian"={"A (VHz)"=0.0, "ω (Hz)"=0.0, "Γ (Hz)"=0.0, "φ (rad)"=0.0, "Q"=0.0, "Norm  Ampl"=0.0, "z∞ (V)"=0.0+0.0i, "4corners"={"z (-pi/2)"=0.0+0.0i, "z(inf)"=0.0+0.0i, "z (pi/2)"=0.0+0.0i, "z center"=0.0+0.0i, "z(0)"=0.0+0.0i, "radius"=0.0}}, "timestamp(min)"=1812.4666666686535, "timestamp"=timestamp(3493836569 s since 1904-01-01), "Magn Field(T)"=0.0}, {"temperature"=27.202, "lorentzian"={"A (VHz)"=0.0, "ω (Hz)"=0.0, "Γ (Hz)"=0.0, "φ (rad)"=0.0, "Q"=0.0, "Norm  Ampl"=0.0, "z∞ (V)"=0.0+0.0i, "4corners"={"z (-pi/2)"=0.0+0.0i, "z(inf)"=0.0+0.0i, "z (pi/2)"=0.0+0.0i, "z center"=0.0+0.0i, "z(0)"=0.0+0.0i, "radius"=0.0}}, "timestamp(min)"=1813.7833333313465, "timestamp"=timestamp(3493836648 s since 1904-01-01), "Magn Field(T)"=0.0}, {"temperature"=27.113, "lorentzian"={"A (VHz)"=0.0, "ω (Hz)"=0.0, "Γ (Hz)"=0.0, "φ (rad)"=0.0, "Q"=0.0, "Norm  Ampl"=0.0, "z∞ (V)"=0.0+0.0i, "4corners"={"z (-pi/2)"=0.0+0.0i, "z(inf)"=0.0+0.0i, "z (pi/2)"=0.0+0.0i, "z center"=0.0+0.0i, "z(0)"=0.0+0.0i, "radius"=0.0}}, "timestamp(min)"=1815.1166666671634, "timestamp"=timestamp(3493836728 s since 1904-01-01), "Magn Field(T)"=0.0}, {"temperature"=27.012, "lorentzian"={"A (VHz)"=0.0, "ω (Hz)"=0.0, "Γ (Hz)"=0.0, "φ (rad)"=0.0, "Q"=0.0, "Norm  Ampl"=0.0, "z∞ (V)"=0.0+0.0i, "4corners"={"z (-pi/2)"=0.0+0.0i, "z(inf)"=0.0+0.0i, "z (pi/2)"=0.0+0.0i, "z center"=0.0+0.0i, "z(0)"=0.0+0.0i, "radius"=0.0}}, "timestamp(min)"=1816.433333337307, "timestamp"=timestamp(3493836807 s since 1904-01-01), "Magn Field(T)"=0.0}, {"temperature"=26.919, "lorentzian"={"A (VHz)"=0.0, "ω (Hz)"=0.0, "Γ (Hz)"=0.0, "φ (rad)"=0.0, "Q"=0.0, "Norm  Ampl"=0.0, "z∞ (V)"=0.0+0.0i, "4corners"={"z (-pi/2)"=0.0+0.0i, "z(inf)"=0.0+0.0i, "z (pi/2)"=0.0+0.0i, "z center"=0.0+0.0i, "z(0)"=0.0+0.0i, "radius"=0.0}}, "timestamp(min)"=1817.75, "timestamp"=timestamp(3493836886 s since 1904-01-01), "Magn Field(T)"=0.0}, {"temperature"=26.829, "lorentzian"={"A (VHz)"=0.0, "ω (Hz)"=0.0, "Γ (Hz)"=0.0, "φ (rad)"=0.0, "Q"=0.0, "Norm  Ampl"=0.0, "z∞ (V)"=0.0+0.0i, "4corners"={"z (-pi/2)"=0.0+0.0i, "z(inf)"=0.0+0.0i, "z (pi/2)"=0.0+0.0i, "z center"=0.0+0.0i, "z(0)"=0.0+0.0i, "radius"=0.0}}, "timestamp(min)"=1819.0833333358169, "timestamp"=timestamp(3493836966 s since 1904-01-01), "Magn Field(T)"=0.0}, {"temperature"=26.729, "lorentzian"={"A (VHz)"=0.0, "ω (Hz)"=0.0, "Γ (Hz)"=0.0, "φ (rad)"=0.0, "Q"=0.0, "Norm  Ampl"=0.0, "z∞ (V)"=0.0+0.0i, "4corners"={"z (-pi/2)"=0.0+0.0i, "z(inf)"=0.0+0.0i, "z (pi/2)"=0.0+0.0i, "z center"=0.0+0.0i, "z(0)"=0.0+0.0i, "radius"=0.0}}, "timestamp(min)"=1820.3999999985099, "timestamp"=timestamp(3493837045 s since 1904-01-01), "Magn Field(T)"=0.0}, {"temperature"=26.631, "lorentzian"={"A (VHz)"=0.0, "ω (Hz)"=0.0, "Γ (Hz)"=0.0, "φ (rad)"=0.0, "Q"=0.0, "Norm  Ampl"=0.0, "z∞ (V)"=0.0+0.0i, "4corners"={"z (-pi/2)"=0.0+0.0i, "z(inf)"=0.0+0.0i, "z (pi/2)"=0.0+0.0i, "z center"=0.0+0.0i, "z(0)"=0.0+0.0i, "radius"=0.0}}, "timestamp(min)"=1821.7166666686535, "timestamp"=timestamp(3493837124 s since 1904-01-01), "Magn Field(T)"=0.0}, {"temperature"=26.532, "lorentzian"={"A (VHz)"=0.0, "ω (Hz)"=0.0, "Γ (Hz)"=0.0, "φ (rad)"=0.0, "Q"=0.0, "Norm  Ampl"=0.0, "z∞ (V)"=0.0+0.0i, "4corners"={"z (-pi/2)"=0.0+0.0i, "z(inf)"=0.0+0.0i, "z (pi/2)"=0.0+0.0i, "z center"=0.0+0.0i, "z(0)"=0.0+0.0i, "radius"=0.0}}, "timestamp(min)"=1823.0500000044703, "timestamp"=timestamp(3493837204 s since 1904-01-01), "Magn Field(T)"=0.0}, {"temperature"=26.444, "lorentzian"={"A (VHz)"=0.0, "ω (Hz)"=0.0, "Γ (Hz)"=0.0, "φ (rad)"=0.0, "Q"=0.0, "Norm  Ampl"=0.0, "z∞ (V)"=0.0+0.0i, "4corners"={"z (-pi/2)"=0.0+0.0i, "z(inf)"=0.0+0.0i, "z (pi/2)"=0.0+0.0i, "z center"=0.0+0.0i, "z(0)"=0.0+0.0i, "radius"=0.0}}, "timestamp(min)"=1824.3666666671634, "timestamp"=timestamp(3493837283 s since 1904-01-01), "Magn Field(T)"=0.0}, {"temperature"=26.344, "lorentzian"={"A (VHz)"=0.0, "ω (Hz)"=0.0, "Γ (Hz)"=0.0, "φ (rad)"=0.0, "Q"=0.0, "Norm  Ampl"=0.0, "z∞ (V)"=0.0+0.0i, "4corners"={"z (-pi/2)"=0.0+0.0i, "z(inf)"=0.0+0.0i, "z (pi/2)"=0.0+0.0i, "z center"=0.0+0.0i, "z(0)"=0.0+0.0i, "radius"=0.0}}, "timestamp(min)"=1825.7000000029802, "timestamp"=timestamp(3493837363 s since 1904-01-01), "Magn Field(T)"=0.0}, {"temperature"=26.256, "lorentzian"={"A (VHz)"=0.0, "ω (Hz)"=0.0, "Γ (Hz)"=0.0, "φ (rad)"=0.0, "Q"=0.0, "Norm  Ampl"=0.0, "z∞ (V)"=0.0+0.0i, "4corners"={"z (-pi/2)"=0.0+0.0i, "z(inf)"=0.0+0.0i, "z (pi/2)"=0.0+0.0i, "z center"=0.0+0.0i, "z(0)"=0.0+0.0i, "radius"=0.0}}, "timestamp(min)"=1827.0166666656733, "timestamp"=timestamp(3493837442 s since 1904-01-01), "Magn Field(T)"=0.0}, {"temperature"=26.156, "lorentzian"={"A (VHz)"=0.0, "ω (Hz)"=0.0, "Γ (Hz)"=0.0, "φ (rad)"=0.0, "Q"=0.0, "Norm  Ampl"=0.0, "z∞ (V)"=0.0+0.0i, "4corners"={"z (-pi/2)"=0.0+0.0i, "z(inf)"=0.0+0.0i, "z (pi/2)"=0.0+0.0i, "z center"=0.0+0.0i, "z(0)"=0.0+0.0i, "radius"=0.0}}, "timestamp(min)"=1828.3333333358169, "timestamp"=timestamp(3493837521 s since 1904-01-01), "Magn Field(T)"=0.0}, {"temperature"=26.051, "lorentzian"={"A (VHz)"=0.0, "ω (Hz)"=0.0, "Γ (Hz)"=0.0, "φ (rad)"=0.0, "Q"=0.0, "Norm  Ampl"=0.0, "z∞ (V)"=0.0+0.0i, "4corners"={"z (-pi/2)"=0.0+0.0i, "z(inf)"=0.0+0.0i, "z (pi/2)"=0.0+0.0i, "z center"=0.0+0.0i, "z(0)"=0.0+0.0i, "radius"=0.0}}, "timestamp(min)"=1829.6666666641831, "timestamp"=timestamp(3493837601 s since 1904-01-01), "Magn Field(T)"=0.0}, {"temperature"=25.961, "lorentzian"={"A (VHz)"=0.0, "ω (Hz)"=0.0, "Γ (Hz)"=0.0, "φ (rad)"=0.0, "Q"=0.0, "Norm  Ampl"=0.0, "z∞ (V)"=0.0+0.0i, "4corners"={"z (-pi/2)"=0.0+0.0i, "z(inf)"=0.0+0.0i, "z (pi/2)"=0.0+0.0i, "z center"=0.0+0.0i, "z(0)"=0.0+0.0i, "radius"=0.0}}, "timestamp(min)"=1830.9833333343267, "timestamp"=timestamp(3493837680 s since 1904-01-01), "Magn Field(T)"=0.0}, {"temperature"=25.864, "lorentzian"={"A (VHz)"=0.0, "ω (Hz)"=0.0, "Γ (Hz)"=0.0, "φ (rad)"=0.0, "Q"=0.0, "Norm  Ampl"=0.0, "z∞ (V)"=0.0+0.0i, "4corners"={"z (-pi/2)"=0.0+0.0i, "z(inf)"=0.0+0.0i, "z (pi/2)"=0.0+0.0i, "z center"=0.0+0.0i, "z(0)"=0.0+0.0i, "radius"=0.0}}, "timestamp(min)"=1832.3166666701436, "timestamp"=timestamp(3493837760 s since 1904-01-01), "Magn Field(T)"=0.0}, {"temperature"=25.765, "lorentzian"={"A (VHz)"=0.0, "ω (Hz)"=0.0, "Γ (Hz)"=0.0, "φ (rad)"=0.0, "Q"=0.0, "Norm  Ampl"=0.0, "z∞ (V)"=0.0+0.0i, "4corners"={"z (-pi/2)"=0.0+0.0i, "z(inf)"=0.0+0.0i, "z (pi/2)"=0.0+0.0i, "z center"=0.0+0.0i, "z(0)"=0.0+0.0i, "radius"=0.0}}, "timestamp(min)"=1833.6333333328366, "timestamp"=timestamp(3493837839 s since 1904-01-01), "Magn Field(T)"=0.0}, {"temperature"=25.672, "lorentzian"={"A (VHz)"=0.0, "ω (Hz)"=0.0, "Γ (Hz)"=0.0, "φ (rad)"=0.0, "Q"=0.0, "Norm  Ampl"=0.0, "z∞ (V)"=0.0+0.0i, "4corners"={"z (-pi/2)"=0.0+0.0i, "z(inf)"=0.0+0.0i, "z (pi/2)"=0.0+0.0i, "z center"=0.0+0.0i, "z(0)"=0.0+0.0i, "radius"=0.0}}, "timestamp(min)"=1834.9500000029802, "timestamp"=timestamp(3493837918 s since 1904-01-01), "Magn Field(T)"=0.0}, {"temperature"=25.576, "lorentzian"={"A (VHz)"=0.0, "ω (Hz)"=0.0, "Γ (Hz)"=0.0, "φ (rad)"=0.0, "Q"=0.0, "Norm  Ampl"=0.0, "z∞ (V)"=0.0+0.0i, "4corners"={"z (-pi/2)"=0.0+0.0i, "z(inf)"=0.0+0.0i, "z (pi/2)"=0.0+0.0i, "z center"=0.0+0.0i, "z(0)"=0.0+0.0i, "radius"=0.0}}, "timestamp(min)"=1836.2833333313465, "timestamp"=timestamp(3493837998 s since 1904-01-01), "Magn Field(T)"=0.0}, {"temperature"=25.474, "lorentzian"={"A (VHz)"=0.0, "ω (Hz)"=0.0, "Γ (Hz)"=0.0, "φ (rad)"=0.0, "Q"=0.0, "Norm  Ampl"=0.0, "z∞ (V)"=0.0+0.0i, "4corners"={"z (-pi/2)"=0.0+0.0i, "z(inf)"=0.0+0.0i, "z (pi/2)"=0.0+0.0i, "z center"=0.0+0.0i, "z(0)"=0.0+0.0i, "radius"=0.0}}, "timestamp(min)"=1837.6000000014901, "timestamp"=timestamp(3493838077 s since 1904-01-01), "Magn Field(T)"=0.0}, {"temperature"=25.388, "lorentzian"={"A (VHz)"=0.0, "ω (Hz)"=0.0, "Γ (Hz)"=0.0, "φ (rad)"=0.0, "Q"=0.0, "Norm  Ampl"=0.0, "z∞ (V)"=0.0+0.0i, "4corners"={"z (-pi/2)"=0.0+0.0i, "z(inf)"=0.0+0.0i, "z (pi/2)"=0.0+0.0i, "z center"=0.0+0.0i, "z(0)"=0.0+0.0i, "radius"=0.0}}, "timestamp(min)"=1838.9166666641831, "timestamp"=timestamp(3493838156 s since 1904-01-01), "Magn Field(T)"=0.0}, {"temperature"=25.289, "lorentzian"={"A (VHz)"=0.0, "ω (Hz)"=0.0, "Γ (Hz)"=0.0, "φ (rad)"=0.0, "Q"=0.0, "Norm  Ampl"=0.0, "z∞ (V)"=0.0+0.0i, "4corners"={"z (-pi/2)"=0.0+0.0i, "z(inf)"=0.0+0.0i, "z (pi/2)"=0.0+0.0i, "z center"=0.0+0.0i, "z(0)"=0.0+0.0i, "radius"=0.0}}, "timestamp(min)"=1840.25, "timestamp"=timestamp(3493838236 s since 1904-01-01), "Magn Field(T)"=0.0}, {"temperature"=25.188, "lorentzian"={"A (VHz)"=0.0, "ω (Hz)"=0.0, "Γ (Hz)"=0.0, "φ (rad)"=0.0, "Q"=0.0, "Norm  Ampl"=0.0, "z∞ (V)"=0.0+0.0i, "4corners"={"z (-pi/2)"=0.0+0.0i, "z(inf)"=0.0+0.0i, "z (pi/2)"=0.0+0.0i, "z center"=0.0+0.0i, "z(0)"=0.0+0.0i, "radius"=0.0}}, "timestamp(min)"=1841.5666666701436, "timestamp"=timestamp(3493838315 s since 1904-01-01), "Magn Field(T)"=0.0}, {"temperature"=25.098, "lorentzian"={"A (VHz)"=0.0, "ω (Hz)"=0.0, "Γ (Hz)"=0.0, "φ (rad)"=0.0, "Q"=0.0, "Norm  Ampl"=0.0, "z∞ (V)"=0.0+0.0i, "4corners"={"z (-pi/2)"=0.0+0.0i, "z(inf)"=0.0+0.0i, "z (pi/2)"=0.0+0.0i, "z center"=0.0+0.0i, "z(0)"=0.0+0.0i, "radius"=0.0}}, "timestamp(min)"=1842.8999999985099, "timestamp"=timestamp(3493838395 s since 1904-01-01), "Magn Field(T)"=0.0}, {"temperature"=24.995, "lorentzian"={"A (VHz)"=0.0, "ω (Hz)"=0.0, "Γ (Hz)"=0.0, "φ (rad)"=0.0, "Q"=0.0, "Norm  Ampl"=0.0, "z∞ (V)"=0.0+0.0i, "4corners"={"z (-pi/2)"=0.0+0.0i, "z(inf)"=0.0+0.0i, "z (pi/2)"=0.0+0.0i, "z center"=0.0+0.0i, "z(0)"=0.0+0.0i, "radius"=0.0}}, "timestamp(min)"=1844.2166666686535, "timestamp"=timestamp(3493838474 s since 1904-01-01), "Magn Field(T)"=0.0}, {"temperature"=24.901, "lorentzian"={"A (VHz)"=0.0, "ω (Hz)"=0.0, "Γ (Hz)"=0.0, "φ (rad)"=0.0, "Q"=0.0, "Norm  Ampl"=0.0, "z∞ (V)"=0.0+0.0i, "4corners"={"z (-pi/2)"=0.0+0.0i, "z(inf)"=0.0+0.0i, "z (pi/2)"=0.0+0.0i, "z center"=0.0+0.0i, "z(0)"=0.0+0.0i, "radius"=0.0}}, "timestamp(min)"=1845.5333333313465, "timestamp"=timestamp(3493838553 s since 1904-01-01), "Magn Field(T)"=0.0}, {"temperature"=24.798, "lorentzian"={"A (VHz)"=0.0, "ω (Hz)"=0.0, "Γ (Hz)"=0.0, "φ (rad)"=0.0, "Q"=0.0, "Norm  Ampl"=0.0, "z∞ (V)"=0.0+0.0i, "4corners"={"z (-pi/2)"=0.0+0.0i, "z(inf)"=0.0+0.0i, "z (pi/2)"=0.0+0.0i, "z center"=0.0+0.0i, "z(0)"=0.0+0.0i, "radius"=0.0}}, "timestamp(min)"=1846.8666666671634, "timestamp"=timestamp(3493838633 s since 1904-01-01), "Magn Field(T)"=0.0}, {"temperature"=24.697, "lorentzian"={"A (VHz)"=0.0, "ω (Hz)"=0.0, "Γ (Hz)"=0.0, "φ (rad)"=0.0, "Q"=0.0, "Norm  Ampl"=0.0, "z∞ (V)"=0.0+0.0i, "4corners"={"z (-pi/2)"=0.0+0.0i, "z(inf)"=0.0+0.0i, "z (pi/2)"=0.0+0.0i, "z center"=0.0+0.0i, "z(0)"=0.0+0.0i, "radius"=0.0}}, "timestamp(min)"=1848.183333337307, "timestamp"=timestamp(3493838712 s since 1904-01-01), "Magn Field(T)"=0.0}, {"temperature"=24.601, "lorentzian"={"A (VHz)"=0.0, "ω (Hz)"=0.0, "Γ (Hz)"=0.0, "φ (rad)"=0.0, "Q"=0.0, "Norm  Ampl"=0.0, "z∞ (V)"=0.0+0.0i, "4corners"={"z (-pi/2)"=0.0+0.0i, "z(inf)"=0.0+0.0i, "z (pi/2)"=0.0+0.0i, "z center"=0.0+0.0i, "z(0)"=0.0+0.0i, "radius"=0.0}}, "timestamp(min)"=1849.5, "timestamp"=timestamp(3493838791 s since 1904-01-01), "Magn Field(T)"=0.0}, {"temperature"=24.516, "lorentzian"={"A (VHz)"=0.0, "ω (Hz)"=0.0, "Γ (Hz)"=0.0, "φ (rad)"=0.0, "Q"=0.0, "Norm  Ampl"=0.0, "z∞ (V)"=0.0+0.0i, "4corners"={"z (-pi/2)"=0.0+0.0i, "z(inf)"=0.0+0.0i, "z (pi/2)"=0.0+0.0i, "z center"=0.0+0.0i, "z(0)"=0.0+0.0i, "radius"=0.0}}, "timestamp(min)"=1850.8333333358169, "timestamp"=timestamp(3493838871 s since 1904-01-01), "Magn Field(T)"=0.0}, {"temperature"=24.408, "lorentzian"={"A (VHz)"=0.0, "ω (Hz)"=0.0, "Γ (Hz)"=0.0, "φ (rad)"=0.0, "Q"=0.0, "Norm  Ampl"=0.0, "z∞ (V)"=0.0+0.0i, "4corners"={"z (-pi/2)"=0.0+0.0i, "z(inf)"=0.0+0.0i, "z (pi/2)"=0.0+0.0i, "z center"=0.0+0.0i, "z(0)"=0.0+0.0i, "radius"=0.0}}, "timestamp(min)"=1852.1499999985099, "timestamp"=timestamp(3493838950 s since 1904-01-01), "Magn Field(T)"=0.0}, {"temperature"=24.313, "lorentzian"={"A (VHz)"=0.0, "ω (Hz)"=0.0, "Γ (Hz)"=0.0, "φ (rad)"=0.0, "Q"=0.0, "Norm  Ampl"=0.0, "z∞ (V)"=0.0+0.0i, "4corners"={"z (-pi/2)"=0.0+0.0i, "z(inf)"=0.0+0.0i, "z (pi/2)"=0.0+0.0i, "z center"=0.0+0.0i, "z(0)"=0.0+0.0i, "radius"=0.0}}, "timestamp(min)"=1853.4833333343267, "timestamp"=timestamp(3493839030 s since 1904-01-01), "Magn Field(T)"=0.0}, {"temperature"=24.219, "lorentzian"={"A (VHz)"=0.0, "ω (Hz)"=0.0, "Γ (Hz)"=0.0, "φ (rad)"=0.0, "Q"=0.0, "Norm  Ampl"=0.0, "z∞ (V)"=0.0+0.0i, "4corners"={"z (-pi/2)"=0.0+0.0i, "z(inf)"=0.0+0.0i, "z (pi/2)"=0.0+0.0i, "z center"=0.0+0.0i, "z(0)"=0.0+0.0i, "radius"=0.0}}, "timestamp(min)"=1854.8000000044703, "timestamp"=timestamp(3493839109 s since 1904-01-01), "Magn Field(T)"=0.0}, {"temperature"=24.112, "lorentzian"={"A (VHz)"=0.0, "ω (Hz)"=0.0, "Γ (Hz)"=0.0, "φ (rad)"=0.0, "Q"=0.0, "Norm  Ampl"=0.0, "z∞ (V)"=0.0+0.0i, "4corners"={"z (-pi/2)"=0.0+0.0i, "z(inf)"=0.0+0.0i, "z (pi/2)"=0.0+0.0i, "z center"=0.0+0.0i, "z(0)"=0.0+0.0i, "radius"=0.0}}, "timestamp(min)"=1856.1166666671634, "timestamp"=timestamp(3493839188 s since 1904-01-01), "Magn Field(T)"=0.0}, {"temperature"=24.023, "lorentzian"={"A (VHz)"=0.0, "ω (Hz)"=0.0, "Γ (Hz)"=0.0, "φ (rad)"=0.0, "Q"=0.0, "Norm  Ampl"=0.0, "z∞ (V)"=0.0+0.0i, "4corners"={"z (-pi/2)"=0.0+0.0i, "z(inf)"=0.0+0.0i, "z (pi/2)"=0.0+0.0i, "z center"=0.0+0.0i, "z(0)"=0.0+0.0i, "radius"=0.0}}, "timestamp(min)"=1857.4500000029802, "timestamp"=timestamp(3493839268 s since 1904-01-01), "Magn Field(T)"=0.0}, {"temperature"=23.922, "lorentzian"={"A (VHz)"=0.0, "ω (Hz)"=0.0, "Γ (Hz)"=0.0, "φ (rad)"=0.0, "Q"=0.0, "Norm  Ampl"=0.0, "z∞ (V)"=0.0+0.0i, "4corners"={"z (-pi/2)"=0.0+0.0i, "z(inf)"=0.0+0.0i, "z (pi/2)"=0.0+0.0i, "z center"=0.0+0.0i, "z(0)"=0.0+0.0i, "radius"=0.0}}, "timestamp(min)"=1858.7666666656733, "timestamp"=timestamp(3493839347 s since 1904-01-01), "Magn Field(T)"=0.0}, {"temperature"=23.825, "lorentzian"={"A (VHz)"=0.0, "ω (Hz)"=0.0, "Γ (Hz)"=0.0, "φ (rad)"=0.0, "Q"=0.0, "Norm  Ampl"=0.0, "z∞ (V)"=0.0+0.0i, "4corners"={"z (-pi/2)"=0.0+0.0i, "z(inf)"=0.0+0.0i, "z (pi/2)"=0.0+0.0i, "z center"=0.0+0.0i, "z(0)"=0.0+0.0i, "radius"=0.0}}, "timestamp(min)"=1860.1000000014901, "timestamp"=timestamp(3493839427 s since 1904-01-01), "Magn Field(T)"=0.0}, {"temperature"=23.731, "lorentzian"={"A (VHz)"=0.0, "ω (Hz)"=0.0, "Γ (Hz)"=0.0, "φ (rad)"=0.0, "Q"=0.0, "Norm  Ampl"=0.0, "z∞ (V)"=0.0+0.0i, "4corners"={"z (-pi/2)"=0.0+0.0i, "z(inf)"=0.0+0.0i, "z (pi/2)"=0.0+0.0i, "z center"=0.0+0.0i, "z(0)"=0.0+0.0i, "radius"=0.0}}, "timestamp(min)"=1861.4166666641831, "timestamp"=timestamp(3493839506 s since 1904-01-01), "Magn Field(T)"=0.0}, {"temperature"=23.634, "lorentzian"={"A (VHz)"=0.0, "ω (Hz)"=0.0, "Γ (Hz)"=0.0, "φ (rad)"=0.0, "Q"=0.0, "Norm  Ampl"=0.0, "z∞ (V)"=0.0+0.0i, "4corners"={"z (-pi/2)"=0.0+0.0i, "z(inf)"=0.0+0.0i, "z (pi/2)"=0.0+0.0i, "z center"=0.0+0.0i, "z(0)"=0.0+0.0i, "radius"=0.0}}, "timestamp(min)"=1862.7333333343267, "timestamp"=timestamp(3493839585 s since 1904-01-01), "Magn Field(T)"=0.0}, {"temperature"=23.53, "lorentzian"={"A (VHz)"=0.0, "ω (Hz)"=0.0, "Γ (Hz)"=0.0, "φ (rad)"=0.0, "Q"=0.0, "Norm  Ampl"=0.0, "z∞ (V)"=0.0+0.0i, "4corners"={"z (-pi/2)"=0.0+0.0i, "z(inf)"=0.0+0.0i, "z (pi/2)"=0.0+0.0i, "z center"=0.0+0.0i, "z(0)"=0.0+0.0i, "radius"=0.0}}, "timestamp(min)"=1864.0666666701436, "timestamp"=timestamp(3493839665 s since 1904-01-01), "Magn Field(T)"=0.0}, {"temperature"=23.436, "lorentzian"={"A (VHz)"=0.0, "ω (Hz)"=0.0, "Γ (Hz)"=0.0, "φ (rad)"=0.0, "Q"=0.0, "Norm  Ampl"=0.0, "z∞ (V)"=0.0+0.0i, "4corners"={"z (-pi/2)"=0.0+0.0i, "z(inf)"=0.0+0.0i, "z (pi/2)"=0.0+0.0i, "z center"=0.0+0.0i, "z(0)"=0.0+0.0i, "radius"=0.0}}, "timestamp(min)"=1865.3833333328366, "timestamp"=timestamp(3493839744 s since 1904-01-01), "Magn Field(T)"=0.0}, {"temperature"=23.334, "lorentzian"={"A (VHz)"=0.0, "ω (Hz)"=0.0, "Γ (Hz)"=0.0, "φ (rad)"=0.0, "Q"=0.0, "Norm  Ampl"=0.0, "z∞ (V)"=0.0+0.0i, "4corners"={"z (-pi/2)"=0.0+0.0i, "z(inf)"=0.0+0.0i, "z (pi/2)"=0.0+0.0i, "z center"=0.0+0.0i, "z(0)"=0.0+0.0i, "radius"=0.0}}, "timestamp(min)"=1866.7000000029802, "timestamp"=timestamp(3493839823 s since 1904-01-01), "Magn Field(T)"=0.0}, {"temperature"=23.235, "lorentzian"={"A (VHz)"=0.0, "ω (Hz)"=0.0, "Γ (Hz)"=0.0, "φ (rad)"=0.0, "Q"=0.0, "Norm  Ampl"=0.0, "z∞ (V)"=0.0+0.0i, "4corners"={"z (-pi/2)"=0.0+0.0i, "z(inf)"=0.0+0.0i, "z (pi/2)"=0.0+0.0i, "z center"=0.0+0.0i, "z(0)"=0.0+0.0i, "radius"=0.0}}, "timestamp(min)"=1868.0333333313465, "timestamp"=timestamp(3493839903 s since 1904-01-01), "Magn Field(T)"=0.0}, {"temperature"=23.139, "lorentzian"={"A (VHz)"=0.0, "ω (Hz)"=0.0, "Γ (Hz)"=0.0, "φ (rad)"=0.0, "Q"=0.0, "Norm  Ampl"=0.0, "z∞ (V)"=0.0+0.0i, "4corners"={"z (-pi/2)"=0.0+0.0i, "z(inf)"=0.0+0.0i, "z (pi/2)"=0.0+0.0i, "z center"=0.0+0.0i, "z(0)"=0.0+0.0i, "radius"=0.0}}, "timestamp(min)"=1869.3500000014901, "timestamp"=timestamp(3493839982 s since 1904-01-01), "Magn Field(T)"=0.0}, {"temperature"=23.041, "lorentzian"={"A (VHz)"=0.0, "ω (Hz)"=0.0, "Γ (Hz)"=0.0, "φ (rad)"=0.0, "Q"=0.0, "Norm  Ampl"=0.0, "z∞ (V)"=0.0+0.0i, "4corners"={"z (-pi/2)"=0.0+0.0i, "z(inf)"=0.0+0.0i, "z (pi/2)"=0.0+0.0i, "z center"=0.0+0.0i, "z(0)"=0.0+0.0i, "radius"=0.0}}, "timestamp(min)"=1870.683333337307, "timestamp"=timestamp(3493840062 s since 1904-01-01), "Magn Field(T)"=0.0}, {"temperature"=22.937, "lorentzian"={"A (VHz)"=0.0, "ω (Hz)"=0.0, "Γ (Hz)"=0.0, "φ (rad)"=0.0, "Q"=0.0, "Norm  Ampl"=0.0, "z∞ (V)"=0.0+0.0i, "4corners"={"z (-pi/2)"=0.0+0.0i, "z(inf)"=0.0+0.0i, "z (pi/2)"=0.0+0.0i, "z center"=0.0+0.0i, "z(0)"=0.0+0.0i, "radius"=0.0}}, "timestamp(min)"=1872.0, "timestamp"=timestamp(3493840141 s since 1904-01-01), "Magn Field(T)"=0.0}, {"temperature"=22.842, "lorentzian"={"A (VHz)"=0.0, "ω (Hz)"=0.0, "Γ (Hz)"=0.0, "φ (rad)"=0.0, "Q"=0.0, "Norm  Ampl"=0.0, "z∞ (V)"=0.0+0.0i, "4corners"={"z (-pi/2)"=0.0+0.0i, "z(inf)"=0.0+0.0i, "z (pi/2)"=0.0+0.0i, "z center"=0.0+0.0i, "z(0)"=0.0+0.0i, "radius"=0.0}}, "timestamp(min)"=1873.3166666701436, "timestamp"=timestamp(3493840220 s since 1904-01-01), "Magn Field(T)"=0.0}, 
